vi "SD Write Rarely.vi"   [LabVIEW 2013]
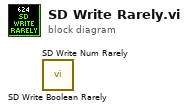
[diagram p0: block diagram]
diagram:
  n1 = call "SD Write Boolean Rarely.vi"() -> ()  [unwired: 12 in]
  n2 = call "SD Write Num Rarely.vi"() -> ()  [unwired: 12 in]
